vi "ReformatAttribute.vi"(7 "format string":string="%s_%d", 8 "error in (no error)":errorcluster, 9 "Attribute default value":string, 10 "Attribute name":string, 11 "Data in":waveform(dbl)[](array[waveform])) -> (0 "error out":errorcluster, 3 "Data out":waveform(dbl)[](array[waveform]))   [LabVIEW 2015]
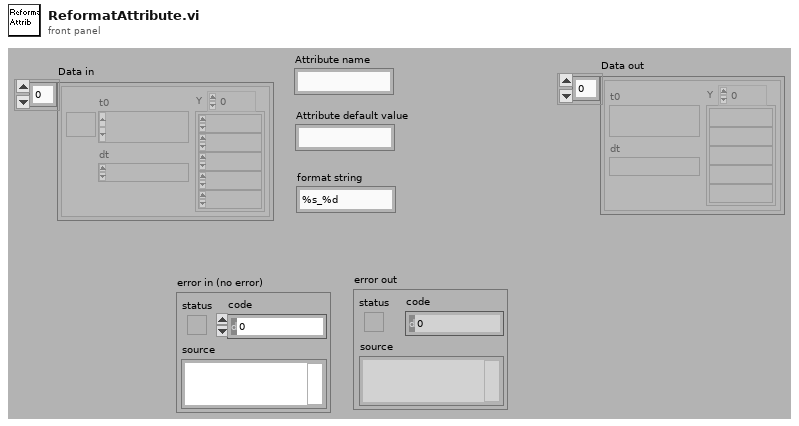
[diagram p1: front panel]
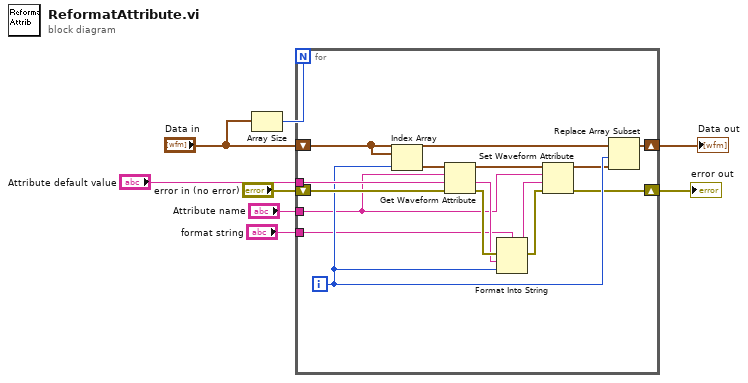
[diagram p0: block diagram]
diagram:
  n1 = Array Size(array="Data in") -> (size(s)=w8:i32)
  n2 = for {
    N: w8 -> [_]
    shift-right: [w22] -> w7
    shift-left: "Data in" -> [w21]
    shift-right: [w13] -> w1
    shift-left: "error in (no error)" -> [w20]
    tunnel: "Attribute name" -> [w12]
    tunnel: "Attribute default value" -> [w19]
    tunnel: "format string" -> [w14]
    i -> [w16]
    n3 = Index Array(array=w21, index=w16) -> (element=w23:waveform(dbl))
    n4 = Get Waveform Attribute(4:w20, 5:w19, 6:w12, 7:w23) -> (0:w18:errorcluster, 1:w15:string, 3:w10:waveform(dbl))  [unwired: 1 out]
    n5 = Format Into String(format string=w14, error in=w18, w15, w16) -> (resulting string=w11:string, error out=w17:errorcluster)  [unwired: 1 in]
    n6 = Set Waveform Attribute(4:w17, 5:w11, 6:w12, 7:w10) -> (0:w13:errorcluster, 3:w9:waveform(dbl))  [unwired: 1 out]
    n7 = Replace Array Subset(array=w21, new element=w9, index=w16) -> (w22:waveform(dbl)[])
  }
  "Data out" <- w7
  "error out" <- w1
